vi "Get CompactSubObj.vi"(8 "error in":errorcluster, 11 "VAR in":refnum<class "VAR.lvclass">) -> (0 "error out":errorcluster, 1 "Set?":bool, 2 "CompactSubObj":u8, 3 "VAR out":refnum<class "VAR.lvclass">)   [LabVIEW 2024, in "Electronic Datasheet.lvlib" / "VAR.lvclass"]
uses:
  VAR.lvclass
  Electronic Datasheet.lvlib
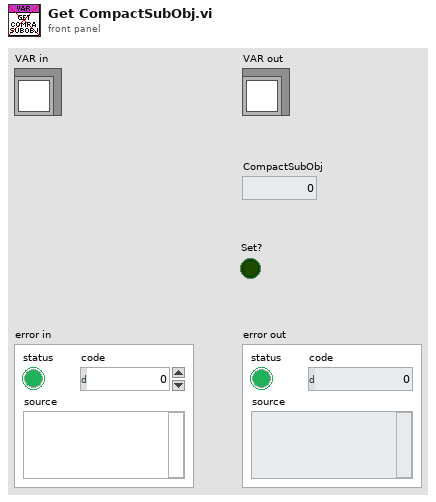
[diagram p1: front panel]
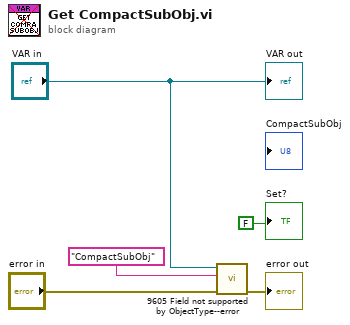
[diagram p0: block diagram]
diagram:
  n1 = call "9605 Field not supported by ObjectType--error.vi"("error in"="error in", "Field Name"="CompactSubObj" ("error message (\"\")"), "Object Type Base"="VAR in") -> ("error out"=→"error out":errorcluster)  [unwired: 8 in]
  "VAR out" <- "VAR in"
  "Set?" <- FALSE ("Set?")
